vi "Inspect.vi"(10 "Msg Strategy in":refnum<class "Msg Strategy.lvclass">=refnum, 11 "TEMPLATE jettl in":refnum<class "TEMPLATE Actor.lvclass">) -> (2 "Msg Strategy out":refnum<class "Msg Strategy.lvclass">, 3 "TEMPLATE jettl out":refnum<class "TEMPLATE Actor.lvclass">)   [LabVIEW 2021, in "_Template.lvlib" / "Templates.lvlib" / "TEMPLATE Actor.lvlib" / "TEMPLATE Actor.lvclass"]
uses:
  TEMPLATE Actor.lvclass
  jettl/jettl/jettl/jettl.lvclass
  jettl/jettl/Msg Strategy/Msg Strategy.lvclass
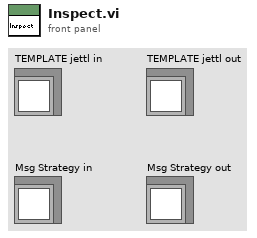
[diagram p1: front panel]
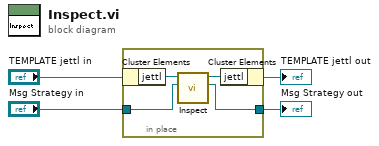
[diagram p0: block diagram]
diagram:
  n1 = in-place {
    in-place-border: "Msg Strategy in" -> [w6]
    in-place-border: [w5] -> w1
    n2 = in-place-cluster #1("TEMPLATE jettl in") -> ("jettl"=w8:refnum<class "jettl.lvclass">)
    n3 = call-dynamic "Inspect.vi"("Msg Strategy in"=w6, "jettl in"=w8) -> ("Msg Strategy out"=w5:refnum<class "Msg Strategy.lvclass">, "jettl out"=w7:refnum<class "jettl.lvclass">)  [unwired: 8 in]
    n4 = in-place-cluster #1("jettl"=w7) -> (→"TEMPLATE jettl out":refnum<class "TEMPLATE Actor.lvclass">)
  }
  "Msg Strategy out" <- w1
